vi "PublishSynchronousRequest.vi"(8 "error in (no error)":errorcluster, 10 "request":T1, 11 "service in":refnum<class "IcmMessageService.lvclass">) -> (0 "error out":errorcluster, 2 "response":T1, 3 "service out":refnum<class "IcmMessageService.lvclass">)   [LabVIEW 2017, in "IcmMessageService.lvclass"]
doc: "Publishes a request message and waits for the response message before returning."
uses:
  <vilib>/addons/InsightCM/MessageBus/MessageService/IcmMessageService.lvclass
  <vilib>/addons/InsightCM/MessageBus/Base/controls/Message.ctl
  <vilib>/addons/InsightCM/MessageBus/Base/controls/MessageHeader.ctl
  <vilib>/addons/InsightCM/MessageBus/Base/controls/KeyValuePair.ctl
  <vilib>/addons/InsightCM/MessageBus/MessageService/IcmMessageService.lvclass/IcmMessageService.ctl
  C:/Program Files (x86)/National Instruments/LabVIEW 2017/vi.lib/addons/InsightCM/Binaries/LabviewMessageAdapter.dll
  Binaries/LabviewMessageAdapter.dll
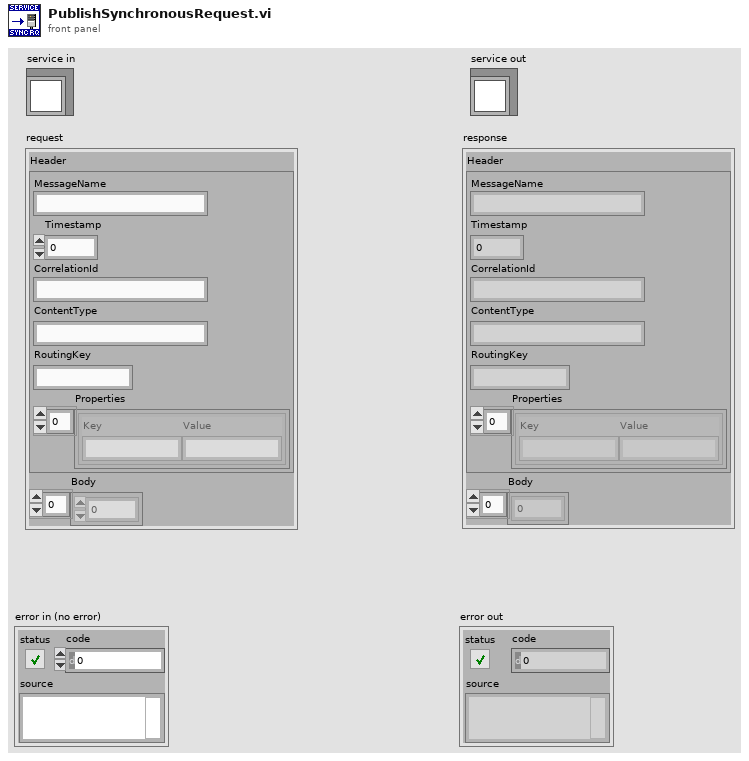
[diagram p1: front panel]
types:
  T1 = typedef "Message.ctl" = cluster{"Header":T2, "Body":u8[]}
  T2 = typedef "MessageHeader.ctl" = cluster{"MessageName":string, "Timestamp":i64, "CorrelationId":string, "ContentType":string, "RoutingKey":string, "Properties":T3[]}
  T3 = typedef "KeyValuePair.ctl" = cluster{"Key":string, "Value":string}
  T4 = typedef "MessageServiceDvr.ctl" = refnum<data-value>
  T5 = typedef "MessageServiceData.ctl" = cluster{"Service":refnum<k24>}
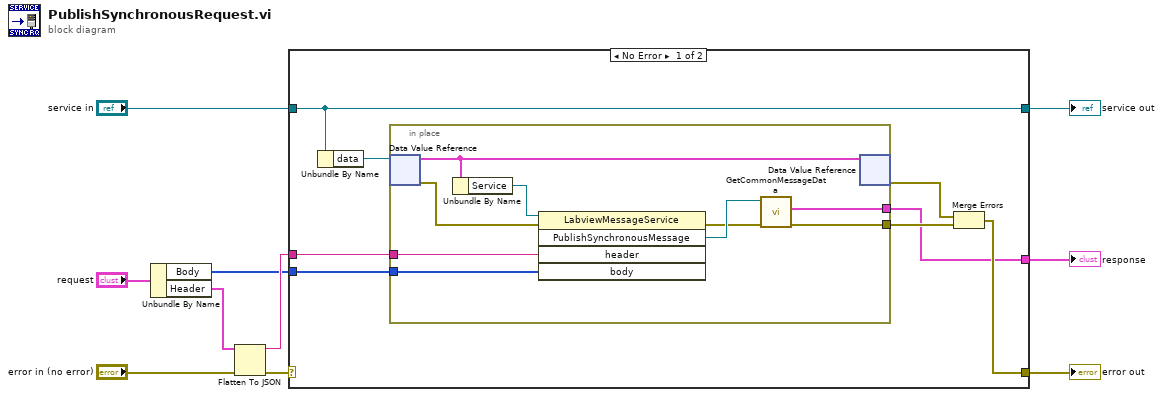
[diagram p0: block diagram]
diagram:
  n1 = Unbundle By Name("request") -> ("Body"=w2:u8[], "Header"=w3:T2)
  n2 = Flatten To JSON(anything=w3, error in (no error)="error in (no error)") -> (JSON string=w5:string, 11:w6:errorcluster)  [unwired: 1 in]
  n3 = case shown="No Error" w6 {
    selector: w6 -> [_ w29]
    tunnel: [w14 w29] -> w10
    tunnel: [w18 w28] -> w8
    tunnel: "service in" -> [w18 w28]
    tunnel: w5 -> [w13 _]
    tunnel: w2 -> [w12 _]
    tunnel: [w11 _] -> w1
    frame No Error {
      n4 = Unbundle By Name(w18) -> ("data"=w17:T4)
      n5 = in-place {
        in-place-border: [w22] -> w15
        in-place-border: w13 -> [w20]
        in-place-border: w12 -> [w19]
        in-place-border: [w21] -> w11
        n6 = in-place-dvr #1(w17) -> (w27:T5, w25:errorcluster)
        n7 = Unbundle By Name(w27) -> ("Service"=w26:refnum<k24>)
        n8 = invoke class="LabviewMessageService" method="PublishSynchronousMessage"(reference=w26, error in=w25, "header"=w20, "body"=w19) -> (error out=w23:errorcluster, "PublishSynchronousMessage"=w24:refnum<k24>)  [unwired: 1 in, 3 out]
        n9 = call <vilib>:"GetCommonMessageData.vi"("error in (no error)"=w23, "MessageArgs"=w24) -> ("error out"=w22:errorcluster, "Message"=w21:T1)  [unwired: 7 in, 1 out]
        n10 = in-place-dvr #1(w27) -> (w16:errorcluster)  [unwired: 1 out]
      }
      n11 = Merge Errors(w16, w15) -> (w14:errorcluster)
    }
    frame Error {
    }
  }
  "error out" <- w10
  "service out" <- w8
  "response" <- w1
